vi "Get Wheel Separations.vi"(8 "error in (no error)":errorcluster, 11 "mecanum steering frame in":refnum<class "NI_Robotics_Mecanum Steering Frame.lvclass">) -> (0 "error out":errorcluster, 1 "wheel separation length":dbl=1.5, 2 "wheel separation width":dbl=1.0, 3 "mecanum steering frame out":refnum<class "NI_Robotics_Mecanum Steering Frame.lvclass">)   [LabVIEW 2017, in "NI_Robotics_Mecanum Steering Frame.lvclass"]
uses:
  <vilib>/robotics/Steering/Mecanum Steering Frame/NI_Robotics_Mecanum Steering Frame.lvclass
  <vilib>/robotics/Steering/Mecanum Steering Frame/NI_Robotics_Mecanum Steering Frame.lvclass/NI_Robotics_Mecanum Steering Frame.ctl
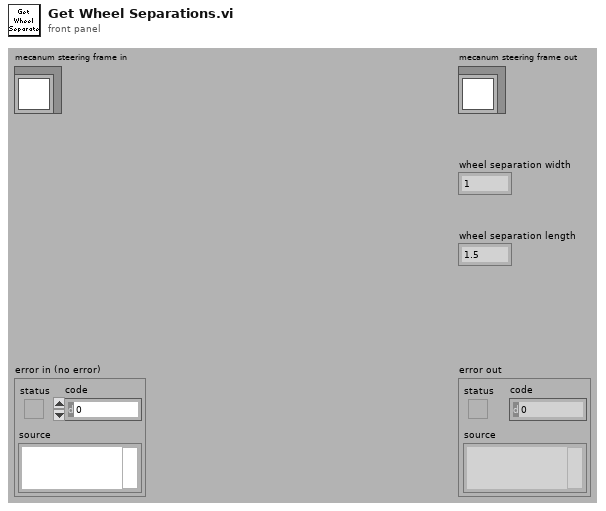
[diagram p1: front panel]
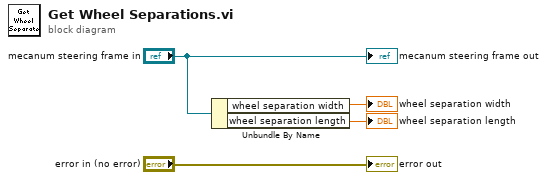
[diagram p0: block diagram]
diagram:
  n1 = Unbundle By Name("mecanum steering frame in") -> ("wheel separation width"=→"wheel separation width":dbl, "wheel separation length"=→"wheel separation length":dbl)
  "error out" <- "error in (no error)"
  "mecanum steering frame out" <- "mecanum steering frame in"
